vi "Start Position.vi"(0 "error in (no error)":errorcluster) -> (1 "function return":i32, 2 "error out":errorcluster)   [LabVIEW 2014, in "ThorZStepper.lvlib"]
doc: "long StartPosition();"
uses:
  ThorZStepper.lvlib
  ThorZStepper.dll
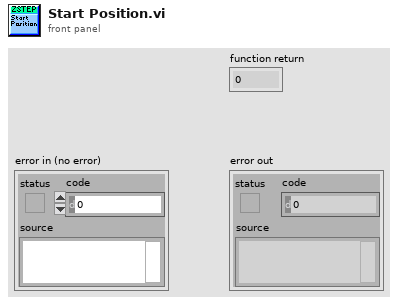
[diagram p1: front panel]
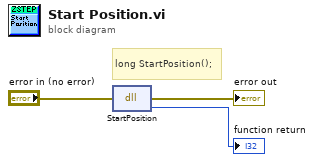
[diagram p0: block diagram]
diagram:
  # "long StartPosition();"
  n1 = dll-call lib="C:/TIS_CalebVS2012/TIS_Development/Hardware/SDKs/MFC1_SDK/LabVIEW/inc/ThorZStepper.*" fn="StartPosition"(error in="error in (no error)") -> (error out=→"error out":errorcluster, →"function return":i32)  [unwired: 2 in, 1 out]
